vi "GetPosition.vi"(8 "error in (no error)":errorcluster, 11 "frame in":refnum<class "frame.lvclass">) -> (0 "error out":errorcluster, 2 "position":cluster{"left":u32, "top":u32}, 3 "frame out":refnum<class "frame.lvclass">)   [LabVIEW 2009, in "frame.lvclass"]
uses:
  frame.lvclass
  frame.lvclass/frame.ctl
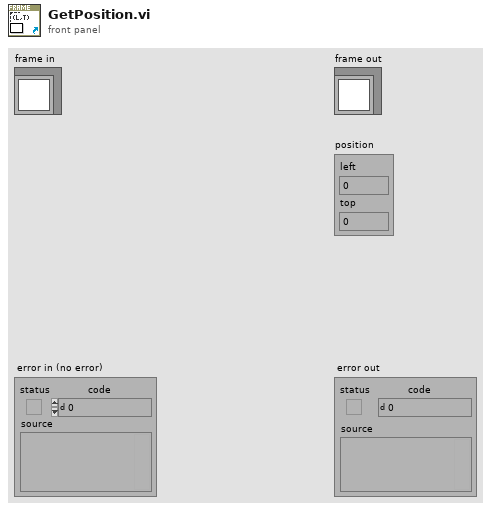
[diagram p1: front panel]
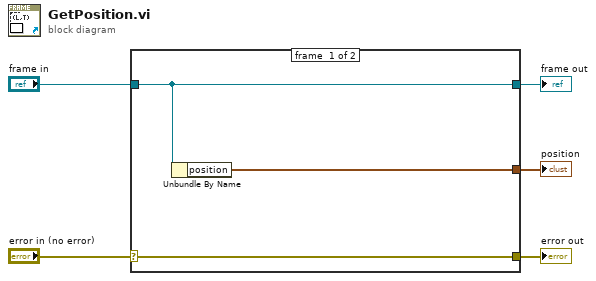
[diagram p0: block diagram]
diagram:
  n1 = case shown="No Error" "error in (no error)" {
    selector: "error in (no error)" -> [w8 w9]
    tunnel: [w8 w9] -> w2
    tunnel: [w7 w10] -> w4
    tunnel: "frame in" -> [w7 w10]
    tunnel: [w6 _] -> w1
    frame #0 {
      n2 = Unbundle By Name(w7) -> ("position"=w6:cluster{"left":u32, "top":u32})
    }
    frame #1 {
    }
  }
  "error out" <- w2
  "frame out" <- w4
  "position" <- w1
